vi "ImagerForFlowbit5_led.vi"() -> ()   [LabVIEW 2011]
uses:
  <vilib>/vision/Image Controls.llb/IMAQ Image.ctl
  <vilib>/Platform/TimedLoop/XDataNode/timing_clust.ctl
  <vilib>/Platform/TimedLoop/XDataNode/nitl_modes.ctl
  <vilib>/Platform/TimedLoop/XDataNode/wakeup.ctl
  <vilib>/Utility/config.llb/Read Key (I32).vi
  <vilib>/Analysis/1siggen.llb/Riffle Array (I32).vi
  <vilib>/Platform/TimedLoop/XDataNode/XDataNode.xnode
  <vilib>/Analysis/NI_AALBase.lvlib
  <vilib>/vision/NI_Vision_Development_Module.lvlib
  <vilib>/Platform/TimedLoop/XDataNode/XDNodeRunTimeDep.lvlib
  <vilib>/Utility/config.llb/NI_LVConfig.lvlib
panel:
  out "onLineMapOutput":T1[](array[typedef])
  out "Bounds.Right":i16
  out "停止循环":bool
  in  "Stimuli":i64=5
  in  "选项卡控件":enum32{"前面板", "参数设置", "OnLineMap"}(tab)
  out "log":string
  out "Stim_ID":i32(listbox)=1
  in  "开始/暂停":bool=TRUE
  in  "停止":bool
  out "重排的 Stim ID":i32[](array[numeric]) caption="重排的{X}"
  out "block":i32
  out "队列中元素数量":i32
  out "Image 2":T1(plugin-control)
  in  "热图":bool
  out "循环持续时间":i64
  out "Recording":bool
  out "grabLoop":i32
  out "writeing data":bool
  out "address":i16=888 caption="地址" format="%.0x"
  in  "SaveParameter":bool
  in  "Pra_binType":enum16{"Extract", "Resample"}(ring)
  in  "Pra_FramesPerStim":i64=16
  in  "Pra_Blk目录":path=path "D:/Expt/test"
  in  "Pra_文件名":string="G4_E02"
  in  "Pra_TimeForPrepare(ms)":u32=1000
  in  "Pra_stim ID":u8[](array[numeric])=[0, 2, 4, 6, 8]
  in  "Pra_blk总数":i32=500
  in  "Pra_stim protocol":T2(array[ring])=[enum."prep stim", enum."wait respirator", enum."show stim", enum."recording data", enum."Blank stim", enum."writing data", enum."ISI"]
  in  "Pra_blank stim":u8
  in  "Pra_wait（ms）":u32=10
  in  "Pra_ISI（ms）":u32=8000
  in  "Pra_FrameBin":i32=25
  in  "Pra_datatype":u16(ring)=13 items=["U8"=11, "I16"=12, "U32"=13, "SGL"=14]
  in  "FrameWidth":i64=704
  in  "FrameHeight":i64=576
  in  "LoadParameter":bool
  in  "Pra_bin":enum16{"1*1", "2*2"}(ring)
  in  "Pra_LED_Current(A)":dbl=0.5 min=0.0001 step=0.1
  in  "Pra_DR/R parameter":T3={"frame_zero_0"=0, "frame_zero_1"=1, "frame_0"=3, "frame_1"=15}
  in  "Pra_OnlineMap":cluster{"数组 1":i32[], "数组 2":i32[]}[](array[cluster])=[{"数组 1"=[2], "数组 2"=[6]}, {"数组 1"=[4], "数组 2"=[8]}, {"数组 1"=[2, 6], "数组 2"=[4, 8]}, {"数组 1"=[2, 4, 6, 8], "数组 2"=[0]}, {"数组 1"=[2, 4], "数组 2"=[6, 8]}]
  in  "Pra_clip ratio":dbl=2.0 min=0.0001 step=0.1
  in  "Pra_LED_COM":refnum<visa-resource-name>="COM3"
  in  "Pra_LED_Max_Voltage(V)":dbl=16.0
  # "-"
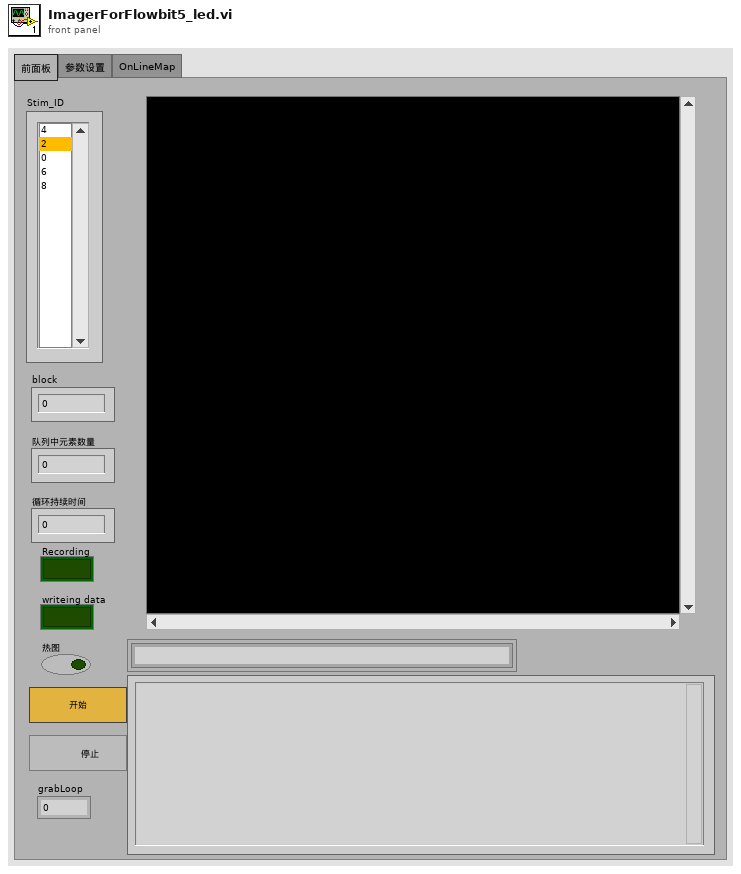
[diagram p1: front panel]
types:
  T1 = typedef "IMAQ Image.ctl" = refnum<image>
  T2 = enum16{"wait", "prep stim", "show stim", "wait respirator", "recording data", "Blank stim", "wait heart", "ISI", "DR/R", "wait calibrate", "openLightShutter", "closeLightShutter", "writing data", "LED on", "LED off"}[]
  T3 = cluster{"frame_zero_0":i32, "frame_zero_1":i32, "frame_0":i32, "frame_1":i32}
  T4 = typedef "Image Type" = u32
  T5 = enum16{"Disable External Trigger", "Enable External Trigger"}
  T6 = enum32{"Auto Detect", "RoadRunner", "Raven", "R64"}
  T7 = typedef "LVAllMonitorsDisplayTypeDef.ctl" = cluster{"Bounds":cluster{"Left":i16, "Top":i16, "Right":i16, "Bottom":i16}, "Depth":i16}[]
  T8 = cluster{"Bounds":cluster{"Left":i16, "Top":i16, "Right":i16, "Bottom":i16}, "Depth":i16}
  T9 = typedef "NI_LVConfig.lvlib/Config Data RefNum.ctl" = refnum<k1>
  T10 = enum16{"big-endian, network order", "native, host order", "little-endian"}
  T11 = enum8{"Enabled", "Disabled", "Disabled and Grayed Out"}
  T12 = enum16{"open", "replace", "create", "open or create", "replace or create", "replace or create with confirmation"}
  T13 = cluster{"Browser Size":cluster{"X":i32, "Y":i32}, "Images per Line":i32, "Background Color":u32, "Frame Size":i32, "Frame Style":enum16{"Raised", "Bevelled", "Outline", "Hidden", "Step", "Raised Outline"}}
  T14 = cluster{"Desired Font (Application)":enum16{"User-specified Font", "Application Font", "System Font", "Dialog Font"}, "[User-specified Font]":cluster{"Font Name":string, "Size":i16, "Strikeout?":bool, "Italic?":bool, "Underline?":bool, "Outline?":bool, "Shadow?":bool, "Bold?":bool, "Rotation Angle":dbl}, "Horizontal Alignment":i16, "Vertical Alignment":i16}
  T15 = typedef "XDNodeRunTimeDep.lvlib/timing_clust.ctl" = cluster{"Expected End [f-1]":u64, "Actual End [f-1]":u64, "Finished Late? [f-1]":bool, "Expected End [i-1]":u64, "Actual End [i-1]":u64, "Finished Late? [i-1]":bool, "Expected Start [i]":u64, "Actual Start [i]":u64, "Expected Start [f]":u64, "Actual Start [f]":u64, "Source Name":string, "Structure Name":string, "Period":i64, "Deadline":i64, "Offset":i64, "Start":i64, "Priority":i32, "Timeout":i32, "Mode":T16, "Wakeup Reason":T17, "Error":errorcluster, "Source Type":string, "Secondary Source Type":string, "Global End Time":u64, "Global Start Time":u64, "Frame Duration":u64, "Iteration Duration":u64, "Assigned CPU":i32, "I/O Scan Engine Mode":u32}
  T16 = typedef "XDNodeRunTimeDep.lvlib/nitl_modes.ctl" = enum32{"No Change", "Process missed periods, maintain original phase", "Discard missed periods, maintain original phase", "Process missed periods, ignore original phase", "Discard missed periods, ignore original phase"}
  T17 = typedef "XDNodeRunTimeDep.lvlib/wakeup.ctl" = enum32{"Normal", "Aborted", "Asynchronous wakeup", "Timing source error", "Timed loop error", "Timeout"}
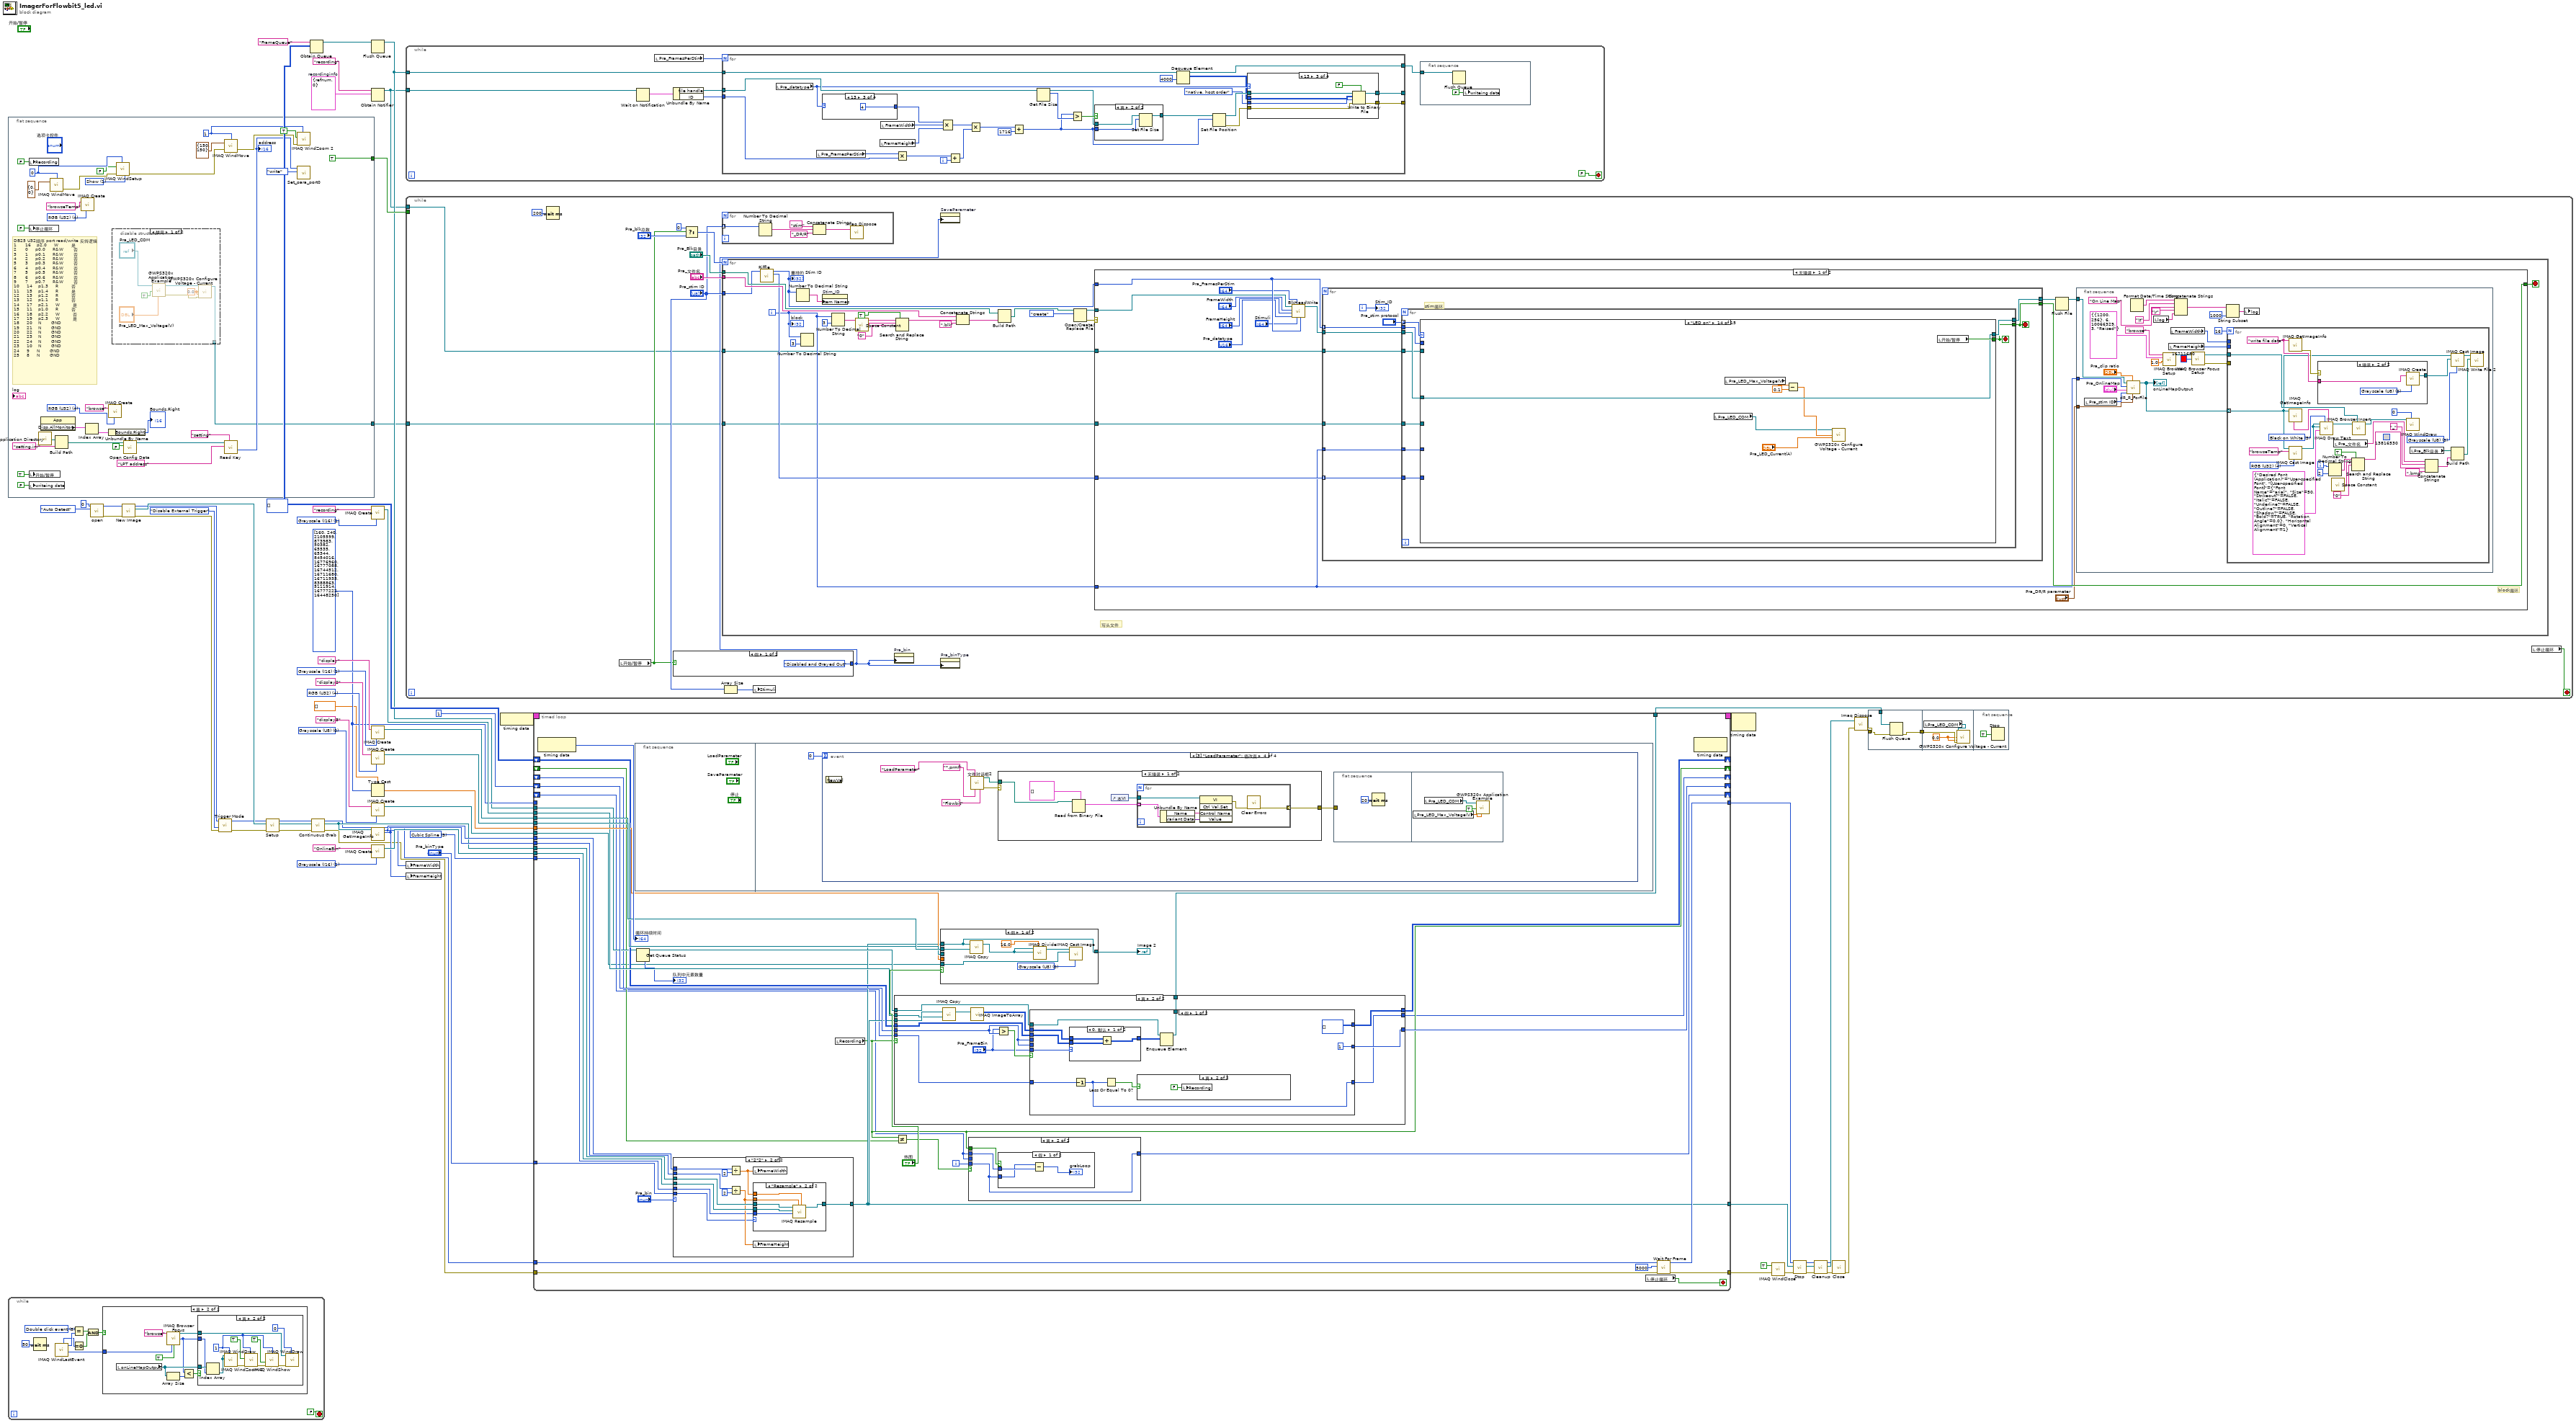
[diagram p0: block diagram]
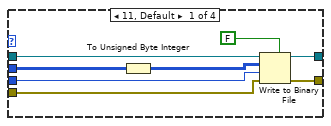
[diagram p4: hidden frame]
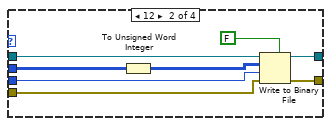
[diagram p5: hidden frame]
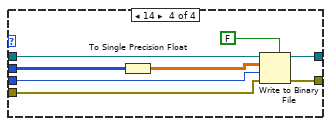
[diagram p6: hidden frame]
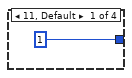
[diagram p8: hidden frame]
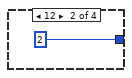
[diagram p9: hidden frame]
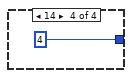
[diagram p10: hidden frame]
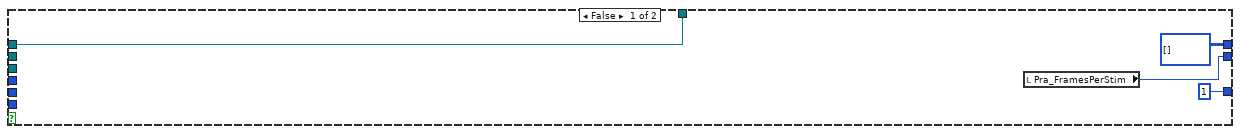
[diagram p11: hidden frame]
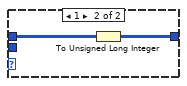
[diagram p13: hidden frame]
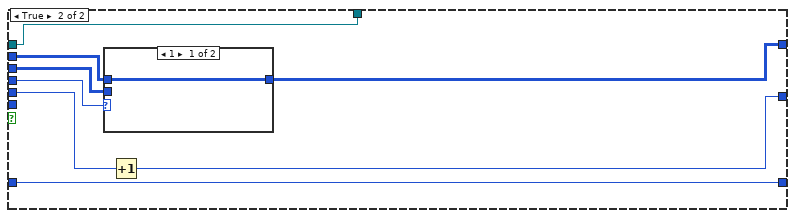
[diagram p14: hidden frame]
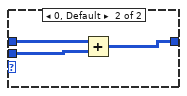
[diagram p15: hidden frame]
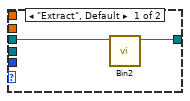
[diagram p19: hidden frame]
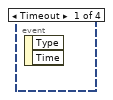
[diagram p20: hidden frame]
diagram:
  w11 = cluster{"file handle":refnum<file>, "ID":i32} {"file handle"=refnum, "ID"=0}  # recordinginfo
  w16 = T4 0 items=["Grayscale (U8)", "Grayscale (I16)", "Grayscale (SGL)", "Complex (CSG)", "RGB (U32)", "HSL (U32)", "RGB (U64)", "Grayscale (U16)"] ("Image Type")
  w21 = u32 3 items=["Zero Order", "Bi-Linear", "Quadratic", "Cubic Spline"] ("Interpolation Type")
  w23 = T4 1 items=["Grayscale (U8)", "Grayscale (I16)", "Grayscale (SGL)", "Complex (CSG)", "RGB (U32)", "HSL (U32)", "RGB (U64)", "Grayscale (U16)"] ("Image Type")
  w25 = u32[][] []
  w34 = T4 4 items=["Grayscale (U8)", "Grayscale (I16)", "Grayscale (SGL)", "Complex (CSG)", "RGB (U32)", "HSL (U32)", "RGB (U64)", "Grayscale (U16)"] ("Image Type")
  w32 = u32[] [160, 240, 2105599, 873983, 50382, 65535, 65344, 8454016, 16776960, 16777088, 16744512, 16711680, 16711935, 8388863, 5111914, 16777222, 16448250] ("数组")
  w38 = T4 1 items=["Grayscale (U8)", "Grayscale (I16)", "Grayscale (SGL)", "Complex (CSG)", "RGB (U32)", "HSL (U32)", "RGB (U64)", "Grayscale (U16)"] ("Image Type")
  w39 = T4 1 items=["Grayscale (U8)", "Grayscale (I16)", "Grayscale (SGL)", "Complex (CSG)", "RGB (U32)", "HSL (U32)", "RGB (U64)", "Grayscale (U16)"] ("Image Type")
  n1 = flat-sequence {
    tunnel: [TRUE ("Zoom to Fit Mode")] -> w27
    tunnel: [w66] -> w4
    frame #0 {
      w72 = 1 items=["Hide", "Show", "No change"] ("Scrollbars (No change)")
      w69 = 1 ("Window Number (0...15)")
      w73 = 0 ("Window Number (0...15)")
      w78 = T4 4 items=["Grayscale (U8)", "Grayscale (I16)", "Grayscale (SGL)", "Complex (CSG)", "RGB (U32)", "HSL (U32)", "RGB (U64)", "Grayscale (U16)"] ("Image Type")
      w79 = T4 4 items=["Grayscale (U8)", "Grayscale (I16)", "Grayscale (SGL)", "Complex (CSG)", "RGB (U32)", "HSL (U32)", "RGB (U64)", "Grayscale (U16)"] ("Image Type")
      # "DB25\tU32顺序\tport\tread/write\t反转逻辑\n1\t     16\t   p2.0    \tW\t        是\n2\t     0    \tp0.0\t   \tR&W\t      否\n3\t     1\t\t   p0.1\t   \tR&W      \t否\n4\t\t    2\t   \tp0.2   \t\tR&W      \t否\n5\t\t    3\t\t   p0.3   \t\tR&W\t      否\n6\t\t    4\t   \tp0.4   \t\tR&W      \t否\n7\t\t    5\t   \tp0.5   \t\tR&W      \t否\n8\t\t    6\t   \tp0.6\t   \tR&W      \t否\n9\t    \t7\t   \tp0.7\t   \tR&W\t      否\n10\t    14   \tp1.3   \t\tR        \t否\n11\t   \t15   \tp1.4   \t\tR        \t是\n12\t   \t13   \tp1.2\t   \tR        \t否\n13    \t12   \tp1.1\t   \tR        \t否\n14     17   \tp2.1\t   \tW        \t是\n15    \t11   \tp1.0   \t\tR\t        否\n16    \t18   \tp2.2   \t\tW        \t否\n17    \t19\t   p2.3   \t\tW\t        是\n18    \t20   \tN   \t  \tGND\t\n19    \t21   \tN   \t  \tGND\t\n20\t    22\t   N\t  \t  \tGND\t\n21\t    23\t   N  \t  \t\tGND\t\n22\t    24\t   N  \t  \t\tGND\t\n23    \t10   \tN  \t  \t\tGND\t\n24    \t9\t    N  \t  \t\tGND\t\n25\t    8    \tN  \t  \t\tGND"
      n2 = local write "Recording"(FALSE ("Recording")) -> ()
      n3 = local write "停止循环"(FALSE ("开始/暂停")) -> ()
      n4 = local write "开始/暂停"(TRUE ("开始/暂停")) -> ()
      n5 = local write "writeing data"(FALSE ("Recording")) -> ()
      n6 = call <vilib>:"Application Directory.vi"() -> ("Application Directory"=w91:path)
      n7 = property class="App"() -> ("Disp.AllMonitors"=w83:T7)  [unwired: 2 in, 2 out]
      n8 = call "IMAQ WindMove"("Window Number (0...15)"=w73, "Coordinates (screen)"=cluster{"X Position":i32, "Y Position":i32} {"X Position"=0, "Y Position"=0}) -> ("error out"=w74:errorcluster)  [unwired: 3 in, 1 out]
      n9 = Build Path(base path=w91, name or relative path="setting.ini" ("名称或相对路径")) -> (appended path=w89:path)
      n10 = call "IMAQ Create"("Image Name"="browseTemp", "Image Type"=w78) -> ()  [unwired: 3 in, 2 out]
      n11 = Index Array(array=w83) -> (element=w82:T8)  [unwired: 1 in]
      n12 = call "IMAQ Create"("Image Name"="browse", "Image Type"=w79) -> ()  [unwired: 3 in, 2 out]
      n13 = Unbundle By Name(w82) -> ("Bounds.Right"=→"Bounds.Right":i16)
      n14 = disable-structure shown="禁用" {
        disable-tunnel: [w100 _] -> w66
        frame Disabled {
          w101 = 0.0 ("Output Voltage (V) (0.0)")
          n15 = call <userlib>:"GWPS320x Application Example.vi"("OVP(V) (0.000)"="Pra_LED_Max_Voltage(V)", "Output State (F:Off)"=TRUE, "VISA session"="Pra_LED_COM") -> ("error out"=w99:errorcluster, "dup VISA session"=w102:refnum<visa-resource-name>)  [unwired: 5 in, 2 out]
          n16 = call <userlib>:"GWPS320x Configure Voltage - Current.vi"("VISA session"=w102, "Output Voltage (V) (0.0)"=w101, "Output Current (A) (0.0)"=w101, "error in (no error)"=w99) -> ("dup VISA session"=w100:refnum<visa-resource-name>)  [unwired: 10 in, 1 out]
        }
        frame Enabled {
        }
      }
      n17 = call "IMAQ WindSetup"("Scrollbars (No change)"=w72, "Window Number (0...15)"=w73, "error in (no error)"=w74, "Window can close? (Yes)"=FALSE) -> ("error out"=w71:errorcluster)  [unwired: 7 in]
      n18 = call <vilib>:"Open Config Data.vi"("create file if necessary (T)"=FALSE, "configuration file path"=w89) -> ("refnum"=w87:T9)  [unwired: 7 in, 2 out]
      n19 = call "IMAQ WindMove"("Window Number (0...15)"=w69, "Coordinates (screen)"=cluster{"X Position":i32, "Y Position":i32} {"X Position"=150, "Y Position"=150}, "error in (no error)"=w71) -> ("error out"=w70:errorcluster)  [unwired: 2 in, 1 out]
      n20 = call-poly <vilib>:"Read Key.vi"("section"="setting", "key"="LPT address", "refnum"=w87) -> ("value"=w84:i32)  [unwired: 5 in, 3 out]
      "address" <- w84
      n21 = call "IMAQ WindZoom 2"("Window Number (0...15)"=w69, "error in (no error)"=w70, "Zoom to Fit? (False)"=TRUE) -> ()  [unwired: 5 in, 4 out]
      n22 = call "Set_para_port0.vi"("R or W"=enum16{"read", "write"}."write", "address"=w84) -> ()  [unwired: 8 in, 2 out]
    }
  }
  n23 = while {
    stop <- FALSE stop-if-true
    w111 = 8 items=["No  event", "Click event", "Draw event", "Move event", "Size event", "Scroll event", "Activate event", "Close event", "Double click event"] ("Event")
    n24 = Wait (ms)(milliseconds to wait=u32 50 ("等待时间（毫秒）")) -> ()  [unwired: 1 out]
    n25 = call "IMAQ WindLastEvent"() -> ("Coordinates"=w105:i32[], "Event"=w110:i32, "Window Number (0...15)"=w109:i32)  [unwired: 6 in, 3 out]
    n26 = Equal?(x=w111, y=w110) -> (x = y?=w108:bool)
    n27 = Equal To 0?(x=w109) -> (x = 0?=w107:bool)
    n28 = And(x=w108, y=w107) -> (x .and. y?=w106:bool)
    n29 = case shown="真" w106 {
      tunnel: w105 -> [_ w121]
      frame False {
      }
      frame True {
        n30 = local read "onLineMapOutput"() -> (w117:T1[])
        n31 = call "IMAQ Browser Focus"("Image Browser In"="browse" ("Image Name"), "Pixel Position"=w121, "Get/Set (Set)"=TRUE) -> ("Image Browser Out"=w115:T1, "Index Out"=w116:i32)  [unwired: 5 in, 6 out]
        n32 = Array Size(array=w117) -> (size(s)=w119:i32)
        n33 = Less?(x=w116, y=w119) -> (x < y?=w118:bool)
        n34 = case shown="真" w118 {
          tunnel: w117 -> [_ w132]
          tunnel: w116 -> [_ w131]
          tunnel: w115 -> [_ w129]
          frame False {
          }
          frame True {
            w123 = 1 ("Window Number (0...15)")
            n35 = Index Array(array=w132, index=w131) -> (element=w130:T1)
            n36 = call "IMAQ WindDraw"("Window Number (0...15)"=w123, "Title"=w130, "Image"=w130) -> ("error out"=w126:errorcluster)  [unwired: 7 in, 1 out]
            n37 = call "IMAQ WindZoom 2"("Window Number (0...15)"=w123, "error in (no error)"=w126, "Zoom to Fit? (False)"=TRUE) -> ("error out"=w125:errorcluster)  [unwired: 5 in, 3 out]
            n38 = call "IMAQ WindShow"("error in (no error)"=w125, "Bring To Front? (N)"=TRUE, "Window Number (0...15)"=w123) -> ("error out"=w124:errorcluster)  [unwired: 3 in, 2 out]
            n39 = call "IMAQ WindDraw"("Window Number (0...15)"=0, "error in (no error)"=w124, "Image"=w129) -> ()  [unwired: 7 in, 2 out]
          }
        }
      }
    }
  }
  n40 = call <vilib>:"open.vi"("Board Type"=T6."Auto Detect", "Board Number"=u32 0) -> ("error out"=w53:errorcluster, "RefBrdOut"=w49:u32)  [unwired: 2 in, 5 out]
  n41 = call <vilib>:"New Image.vi"("RefBrdIn"=w49, "error in"=w53) -> ("RefBrdOut"=w48:u32, "Image"=w61:T1, "error out"=w54:errorcluster)  [unwired: 6 in]
  n42 = call <vilib>:"Trigger Mode.vi"("RefBrdIn"=w48, "Trigger Mode"=T5."Disable External Trigger", "error in (no error)"=w54) -> ("RefBrdOut"=w47:u32, "error out"=w55:errorcluster)  [unwired: 6 in]
  n43 = call <vilib>:"Setup.vi"("error in"=w55, "Image In"=w61, "RefBrdIn"=w47) -> ("error out"=w50:errorcluster, "Image"=w51:T1, "RefBrdOut"=w46:u32)  [unwired: 6 in]
  n44 = Obtain Queue(name (unnamed)="FrameQueue" ("名称（未命名）"), element data type=w25) -> (queue out=w28:refnum<queue>)  [unwired: 3 in, 2 out]
  n45 = call <vilib>:"Continuous Grab.vi"("error in (no error)"=w50, "Image In"=w51, "RefBrdIn"=w46) -> ("error out"=w5:errorcluster, "Image"=w17:T1, "RefBrdOut"=w6:u32)  [unwired: 6 in]
  n46 = Flush Queue(queue=w28) -> (queue out=w13:refnum<queue>)  [unwired: 1 in, 2 out]
  n47 = Obtain Notifier(name (unnamed)="recording" ("名称（未命名）"), notification data type=w11) -> (notifier out=w10:refnum<notifier>)  [unwired: 2 in, 2 out]
  n48 = call "IMAQ Create"("Image Name"="recording", "Image Type"=w39) -> ("New Image"=w41:T1)  [unwired: 3 in, 1 out]
  n49 = call "IMAQ Create"("Image Name"="display", "Image Type"=w38) -> ("New Image"=w36:T1)  [unwired: 3 in, 1 out]
  n50 = call "IMAQ Create"("Image Name"="display2", "Image Type"=w34) -> ("New Image"=w33:T1)  [unwired: 3 in, 1 out]
  n51 = Type Cast(type=sgl[] [] ("单精度浮点"), x=w32) -> (*(type *) &x=w30:sgl[])
  n52 = call "IMAQ Create"("Image Name"="display3", "Image Type"=w16) -> ("New Image"=w14:T1)  [unwired: 3 in, 1 out]
  n53 = call "IMAQ GetImageInfo"("Image"=w17) -> ("Y Resolution"=w19:i32, "X Resolution"=w20:i32)  [unwired: 3 in, 6 out]
  n54 = call "IMAQ Create"("Image Name"="OnlineBin", "Image Type"=w23) -> ("New Image"=w22:T1)  [unwired: 3 in, 1 out]
  n55 = while {
    tunnel: w13 -> [w139]
    tunnel: w10 -> [w137]
    stop <- FALSE stop-if-true
    n56 = Wait on Notification(notifier=w137) -> (notification=w136:cluster{"file handle":refnum<file>, "ID":i32})  [unwired: 3 in, 3 out]
    n57 = local read "Pra_FramesPerStim"() -> (w138:i64)
    n58 = Unbundle By Name(w136) -> ("file handle"=w135:refnum<file>, "ID"=w134:i32)
    n59 = for {
      N: w138 -> [_]
      tunnel: w135 -> [w169]
      tunnel: w134 -> [w153]
      tunnel: [w161] -> _
      tunnel: [w160] -> w133
      tunnel: w139 -> [w145]
      tunnel: [w143] -> _
      i -> [w151]
      n60 = local read "Pra_datatype"() -> (w165:u16)
      n61 = local read "Pra_FramesPerStim"() -> (w154:i64)
      n62 = case shown="13" w165 {
        tunnel: [i64 1 i64 2 i64 4 i64 4] -> w157
        frame 11, Default {
        }
        frame 12 {
        }
        frame 13 {
        }
        frame 14 {
        }
      }
      n63 = local read "FrameHeight"() -> (w155:i64)
      n64 = local read "FrameWidth"() -> (w156:i64)
      n65 = Multiply(x=w154, y=w153) -> (x*y=w152:i64)
      n66 = Compound Arithmetic op=MULTIPLY(w157, w156, w155) -> (w149:i64)
      n67 = Add(x=w152, y=w151) -> (x+y=w150:i64)
      n68 = Multiply(x=w149, y=w150) -> (x*y=w148:i64)
      n69 = Add(x=w148, y=i64 1716 ("x")) -> (x+y=w146:i64)
      n70 = Get File Size(file=w169) -> (refnum out=w162:refnum<file>, size (in bytes)=w158:i64)  [unwired: 1 in, 1 out]
      n71 = Greater?(x=w146, y=w158) -> (0:w163:bool)
      n72 = case shown="真" w163 {
        tunnel: w146 -> [_ w204]
        tunnel: w162 -> [w201 w203]
        tunnel: [w201 w202] -> w164
        frame False {
        }
        frame True {
          n73 = Set File Size(6:w204, 7:w203) -> (3:w202:refnum<file>)  [unwired: 1 in, 1 out]
        }
      }
      n74 = Dequeue Element(queue=w145, timeout in ms (-1)=4000 ("超时毫秒(-1)")) -> (queue out=w160:refnum<queue>, element=w144:u32[][])  [unwired: 1 in, 2 out]
      n75 = Set File Position(offset (in bytes) (0)=w146, refnum=w164) -> (refnum out=w168:refnum<file>, error out=w166:errorcluster)  [unwired: 2 in]
      n76 = case shown="13" w165 {
        tunnel: w144 -> [w172 w181 w187 w194]
        tunnel: w168 -> [w176 w182 w190 w196]
        tunnel: T10."native, host order" ("字节顺序(0:big-endian, network order)") -> [w175 w183 w188 w197]
        tunnel: w166 -> [w174 w178 w189 w198]
        tunnel: [w173 w184 w191 w199] -> w161
        tunnel: [w170 w179 w186 w193] -> w143
        frame 11, Default {
          n77 = To Unsigned Byte Integer(number=w172) -> (unsigned 8bit integer=w171:u8[][])
          n78 = Write to Binary File(file (use dialog)=w176, data=w171, error in=w174, 5:FALSE ("预置数组或字符串大小？(T)"), 9:w175) -> (refnum out=w173:refnum<file>, error out=w170:errorcluster)  [unwired: 1 in, 1 out]
        }
        frame 12 {
          n79 = To Unsigned Word Integer(number=w181) -> (unsigned 16bit integer=w180:u16[][])
          n80 = Write to Binary File(file (use dialog)=w182, data=w180, error in=w178, 5:FALSE ("预置数组或字符串大小？(T)"), 9:w183) -> (refnum out=w184:refnum<file>, error out=w179:errorcluster)  [unwired: 1 in, 1 out]
        }
        frame 13 {
          n81 = Write to Binary File(file (use dialog)=w190, data=w187, error in=w189, 5:FALSE ("预置数组或字符串大小？(T)"), 9:w188) -> (refnum out=w191:refnum<file>, error out=w186:errorcluster)  [unwired: 1 in, 1 out]
        }
        frame 14 {
          n82 = To Single Precision Float(number=w194) -> (single precision float=w195:sgl[][])
          n83 = Write to Binary File(file (use dialog)=w196, data=w195, error in=w198, 5:FALSE ("预置数组或字符串大小？(T)"), 9:w197) -> (refnum out=w199:refnum<file>, error out=w193:errorcluster)  [unwired: 1 in, 1 out]
        }
      }
    }
    n84 = flat-sequence {
      tunnel: w133 -> [w142]
      frame #0 {
        n85 = Flush Queue(queue=w142) -> ()  [unwired: 1 in, 3 out]
        n86 = local write "writeing data"(FALSE ("writeing data")) -> ()
      }
    }
  }
  n87 = while {
    tunnel: w27 -> [_]
    tunnel: w10 -> [w210]
    tunnel: w4 -> [w209]
    stop <- w220 stop-if-true
    n88 = Wait (ms)(milliseconds to wait=u32 200 ("等待时间（毫秒）")) -> ()  [unwired: 1 out]
    n89 = local read "开始/暂停"() -> (w212:bool)
    n90 = case shown="假" w212 {
      tunnel: [T11."Disabled and Grayed Out" ("禁用") T11."Enabled" ("禁用")] -> w211
      frame False {
      }
      frame True {
      }
    }
    n91 = Select(t=0, s=w212, f="Pra_blk总数") -> (s? t:f=w217:i32)
    n92 = for {
      tunnel: "Pra_stim ID" -> [w225] mode=indexing
      n93 = Number To Decimal String(number=w225) -> (decimal integer string=w226:string)  [unwired: 1 in]
      n94 = Concatenate Strings("stim" ("字符串"), w226, "_DR/R" ("字符串")) -> (w224:string)
      n95 = call "Imaq Dispose"("Image"=w224) -> ()  [unwired: 5 in, 1 out]
    }
    n96 = for {
      N: w217 -> [_]
      tunnel: "Pra_stim ID" -> [w247]
      tunnel: "Pra_文件名" -> [w251]
      tunnel: "Pra_Blk目录" -> [w250]
      tunnel: w210 -> [w243]
      tunnel: w209 -> [w229]
      i -> [w245]
      stop <- w248 stop-if-true
      # "写头文件"
      n97 = call-poly <vilib>:"Riffle.vi"("X"=w247) -> ("Riffled Index"=w246:i32[], "Riffled {X}"=w249:i32[])  [unwired: 8 in, 1 out]
      "重排的 Stim ID" <- w249
      n98 = Number To Decimal String(number=w249) -> (decimal integer string=w233:string[])  [unwired: 1 in]
      n99 = Number To Decimal String(number=w245, width (-)=i16 3 ("宽度(-)")) -> ()  [unwired: 1 out]
      n100 = property on="Stim_ID" class="LstBox (严格)"("Item Names"=w233) -> ()  [unwired: 2 in, 2 out]
      n101 = Number To Decimal String(number=w245, width (-)=i16 3 ("宽度(-)")) -> (decimal integer string=w238:string)
      n102 = call <vilib>:"Space Constant.vi"() -> ("String"=w239:string)
      n103 = Search and Replace String(replace all?=TRUE ("替换全部？(F)"), input string=w238, search string=w239, replace string="0" ("替换字符串(\"\")")) -> (result string=w236:string)  [unwired: 4 in, 3 out]
      n104 = Concatenate Strings(w251, w236, ".blk" ("字符串")) -> (w234:string)
      n105 = Build Path(base path=w250, name or relative path=w234) -> (appended path=w244:path)
      n106 = Open/Create/Replace File(file path (use dialog)=w244, operation (0:open)=T12."create" ("操作(0:open)")) -> (refnum out=w231:refnum<file>, error out=w230:errorcluster)  [unwired: 4 in, 1 out]
      n107 = case shown="无错误" w230 {
        tunnel: w249 -> [w266 _]
        tunnel: [w265 TRUE ("开始/暂停")] -> w248
        tunnel: w246 -> [w264 _]
        tunnel: w245 -> [w262 _]
        tunnel: w243 -> [w259 _]
        tunnel: w231 -> [w254 _]
        tunnel: w229 -> [w252 _]
        frame No Error {
          # "block循环"
          n108 = call "BlkHeadWrite.vi"("SequenceOfID"=w266, "Stimuli"="Stimuli", "FramesPerStim"="Pra_FramesPerStim", "datatype"="Pra_datatype", "FrameHeight"="FrameHeight", "FrameWidth"="FrameWidth", "引用句柄输入"=w254) -> ("引用句柄输出"=w267:refnum<file>)  [unwired: 4 in]
          n109 = for {
            tunnel: w267 -> [w335]
            tunnel: [w333] -> w261
            tunnel: w264 -> [w334] mode=indexing
            tunnel: w266 -> [w332] mode=indexing
            tunnel: [w331] -> w265
            tunnel: w262 -> [w328]
            tunnel: w259 -> [w327]
            tunnel: w252 -> [w326]
            i -> [w330]
            stop <- w331 stop-if-true
            # "stim循环"
            n110 = for {
              tunnel: w334 -> [w343]
              tunnel: w332 -> [w341]
              tunnel: [w339] -> w331
              tunnel: "Pra_stim protocol" -> [w340] mode=indexing
              tunnel: w335 -> [w344]
              tunnel: [w342] -> w333
              tunnel: w328 -> [w338]
              tunnel: w327 -> [w337]
              tunnel: w326 -> [w336]
              stop <- w339 stop-if-true
              n111 = case shown="\"LED on\"" w340 {
                tunnel: w344 -> [w347 w367 w382 w396 w413 w426 w440 w455 w477 w487 w489 w502 w515 w531 w539]
                tunnel: w343 -> [_ _ _ w398 _ _ _ w453 _ _ _ _ _ _ _]
                tunnel: [w347 w367 w382 w396 w413 w426 w440 w455 w477 w487 w489 w502 w515 w531 w539] -> w342
                tunnel: w341 -> [w345 _ _ _ _ _ _ _ _ _ _ _ _ _ _]
                tunnel: [w348 w368 w383 w395 w414 w427 w441 w454 w478 w488 w490 w503 w516 w532 w540] -> w339
                tunnel: w338 -> [_ _ _ _ _ _ _ w452 _ _ _ _ _ _ _]
                tunnel: w337 -> [_ _ _ w399 _ _ _ _ _ _ _ _ _ _ _]
                tunnel: w336 -> [_ _ _ _ _ _ _ _ _ _ _ _ _ _ w534]
                frame "prep stim" {
                  n112 = Number To Boolean Array(number=w345) -> (Boolean array=w349:bool[])
                  n113 = flat-sequence {
                    tunnel: w349 -> [w360]
                    tunnel: [w360] -> w346
                    tunnel: w345 -> [w359]
                    tunnel: w346 -> [w365]
                    frame #0 {
                      n114 = Number To Decimal String(number=w359) -> (decimal integer string=w356:string)  [unwired: 1 in]
                      n115 = Format Date/Time String() -> (date/time string=w358:string)  [unwired: 3 in]
                      n116 = local read "log"() -> (w352:string)
                      n117 = Concatenate Strings(w358, "\t", "prep stim ID=" ("字符串"), w356, "\r", w352) -> (w354:string)
                      n118 = String Subset(string=w354, length (rest)=1000 ("y")) -> (substring=w353:string)  [unwired: 1 in]
                      n119 = local write "log"(w353) -> ()
                    }
                    frame #1 {
                      n120 = local read "address"() -> (w362:i16)
                      n121 = local read "address"() -> (w361:i16)
                      n122 = call "Write_para_port0.vi"("port0（8元素）"=w365, "address"=w361) -> ()  [unwired: 9 in, 1 out]
                      n123 = call "Write_para_port2_singalChange.vi"("索引"=0, "布尔"=TRUE, "address"=w362) -> ()  [unwired: 8 in, 1 out]
                    }
                    frame #2 {
                      n124 = Wait (ms)(milliseconds to wait="Pra_TimeForPrepare(ms)") -> ()  [unwired: 1 out]
                    }
                  }
                  n125 = local read "开始/暂停"() -> (w348:bool)
                }
                frame "wait respirator" {
                  n126 = while {
                    stop <- w379 stop-if-true
                    # "this step will return true if pallel port doesn't connect any signal.That means this loop only run once."
                    n127 = Wait (ms)(milliseconds to wait=u32 5 ("等待时间（毫秒）")) -> ()  [unwired: 1 out]
                    n128 = local read "address"() -> (w377:i16)
                    n129 = call "read_para_port1.vi"("address"=w377) -> ("port1（5元素）"=w381:bool[])  [unwired: 9 in, 1 out]
                    n130 = Index Array(array=w381, index=3 ("索引")) -> (element=w379:bool)
                  }
                  n131 = flat-sequence {
                    frame #0 {
                      n132 = Format Date/Time String() -> (date/time string=w376:string)  [unwired: 3 in]
                      n133 = local read "log"() -> (w371:string)
                      n134 = Concatenate Strings(w376, "\t", "wait respiratory" ("字符串"), "\r", w371) -> (w373:string)
                      n135 = String Subset(string=w373, length (rest)=1000 ("y")) -> (substring=w372:string)  [unwired: 1 in]
                      n136 = local write "log"(w372) -> ()
                    }
                  }
                  n137 = local read "开始/暂停"() -> (w368:bool)
                }
                frame "show stim" {
                  n138 = flat-sequence {
                    frame #0 {
                      n139 = local read "address"() -> (w392:i16)
                      n140 = call "Write_para_port2_singalChange.vi"("索引"=0, "布尔"=FALSE, "address"=w392) -> ()  [unwired: 8 in, 1 out]
                    }
                  }
                  n141 = flat-sequence {
                    frame #0 {
                      n142 = Format Date/Time String() -> (date/time string=w391:string)  [unwired: 3 in]
                      n143 = local read "log"() -> (w386:string)
                      n144 = Concatenate Strings(w391, "\t", "show stim" ("字符串"), "\r", w386) -> (w388:string)
                      n145 = String Subset(string=w388, length (rest)=1000 ("y")) -> (substring=w387:string)  [unwired: 1 in]
                      n146 = local write "log"(w387) -> ()
                    }
                  }
                  n147 = local read "开始/暂停"() -> (w383:bool)
                }
                frame "recording data" {
                  n148 = flat-sequence {
                    frame #0 {
                      n149 = Format Date/Time String() -> (date/time string=w411:string)  [unwired: 3 in]
                      n150 = local read "log"() -> (w406:string)
                      n151 = Concatenate Strings(w411, "\t", "recording data" ("字符串"), "\r", w406) -> (w408:string)
                      n152 = String Subset(string=w408, length (rest)=1000 ("y")) -> (substring=w407:string)  [unwired: 1 in]
                      n153 = local write "log"(w407) -> ()
                    }
                  }
                  n154 = flat-sequence {
                    frame #0 {
                      "Recording" <- TRUE ("Recording")
                      "writeing data" <- TRUE ("Recording")
                    }
                    frame #1 {
                      n155 = while {
                        stop <- w403 continue-if-true
                        n156 = local read "Recording"() -> (w403:bool)
                        n157 = Wait (ms)(milliseconds to wait=u32 1 ("等待时间（毫秒）")) -> ()  [unwired: 1 out]
                      }
                    }
                  }
                  n158 = Bundle("引用句柄输出"=w396, w398) -> (w397:cluster{"引用句柄输出":refnum<file>, i32})  [unwired: 1 in]
                  n159 = Send Notification(notification=w397, notifier=w399) -> ()  [unwired: 1 in, 2 out]
                  n160 = local read "开始/暂停"() -> (w395:bool)
                }
                frame "Blank stim" {
                  n161 = flat-sequence {
                    frame #0 {
                      n162 = Format Date/Time String() -> (date/time string=w424:string)  [unwired: 3 in]
                      n163 = local read "log"() -> (w419:string)
                      n164 = Concatenate Strings(w424, "\t", "show blank stim" ("字符串"), "\r", w419) -> (w421:string)
                      n165 = String Subset(string=w421, length (rest)=1000 ("y")) -> (substring=w420:string)  [unwired: 1 in]
                      n166 = local write "log"(w420) -> ()
                    }
                  }
                  n167 = local read "address"() -> (w412:i16)
                  n168 = Number To Boolean Array(number="Pra_blank stim") -> (Boolean array=w415:bool[])
                  n169 = call "Write_para_port0.vi"("port0（8元素）"=w415, "address"=w412) -> ()  [unwired: 9 in, 1 out]
                  n170 = local read "开始/暂停"() -> (w414:bool)
                }
                frame "ISI" {
                  n171 = flat-sequence {
                    tunnel: "Pra_ISI（ms）" -> [w431]
                    tunnel: "Pra_ISI（ms）" -> [w438]
                    frame #0 {
                      n172 = Number To Decimal String(number=w431) -> (decimal integer string=w435:string)  [unwired: 1 in]
                      n173 = Format Date/Time String() -> (date/time string=w437:string)  [unwired: 3 in]
                      n174 = local read "log"() -> (w430:string)
                      n175 = Concatenate Strings(w437, "\t", "ISI(ms)=" ("字符串"), w435, "\r", w430) -> (w433:string)
                      n176 = String Subset(string=w433, length (rest)=1000 ("y")) -> (substring=w432:string)  [unwired: 1 in]
                      n177 = local write "log"(w432) -> ()
                    }
                    frame #1 {
                      n178 = Wait (ms)(milliseconds to wait=w438) -> ()  [unwired: 1 out]
                    }
                  }
                  n179 = local read "开始/暂停"() -> (w427:bool)
                }
                frame "wait", Default {
                  n180 = Wait (ms)(milliseconds to wait="Pra_wait（ms）") -> ()  [unwired: 1 out]
                  n181 = flat-sequence {
                    tunnel: "Pra_wait（ms）" -> [w445]
                    frame #0 {
                      n182 = Number To Decimal String(number=w445) -> (decimal integer string=w449:string)  [unwired: 1 in]
                      n183 = Format Date/Time String() -> (date/time string=w451:string)  [unwired: 3 in]
                      n184 = local read "log"() -> (w444:string)
                      n185 = Concatenate Strings(w451, "\t", "wait(ms)=" ("字符串"), w449, "\r", w444) -> (w447:string)
                      n186 = String Subset(string=w447, length (rest)=1000 ("y")) -> (substring=w446:string)  [unwired: 1 in]
                      n187 = local write "log"(w446) -> ()
                    }
                  }
                  n188 = local read "开始/暂停"() -> (w441:bool)
                }
                frame "DR/R" {
                  n189 = disable-structure shown="禁用" {
                    frame Disabled {
                      n190 = flat-sequence {
                        frame #0 {
                          n191 = Format Date/Time String() -> (date/time string=w463:string)  [unwired: 3 in]
                          n192 = local read "log"() -> (w458:string)
                          n193 = Concatenate Strings(w463, "\t", "DR/R" ("字符串"), "\r", w458) -> (w460:string)
                          n194 = String Subset(string=w460, length (rest)=1000 ("y")) -> (substring=w459:string)  [unwired: 1 in]
                          n195 = local write "log"(w459) -> ()
                        }
                      }
                    }
                    frame Enabled {
                    }
                  }
                  n196 = disable-structure shown="禁用" {
                    disable-tunnel: w453 -> [w468 _]
                    disable-tunnel: w452 -> [w467 _]
                    frame Disabled {
                      n197 = local read item#-1() -> (w464)
                      n198 = Index Array(array=w464, index=w468) -> (element=w465)
                      n199 = call "dR.vi"() -> ("Image Dst Out"=w466:T1)  [unwired: 11 in]
                      n200 = case shown="0" w467 {
                        selector: w467 -> [_ w473]
                        tunnel: w466 -> [w470 w474]
                        tunnel: w465 -> [w469 w476]
                        frame 0 {
                          n201 = call "IMAQ Copy"("Image Dst"=w469, "Image Src"=w470) -> ()  [unwired: 4 in, 2 out]
                        }
                        frame 1, Default {
                          n202 = Increment(x=w473) -> (x+1=w472:i32)
                          n203 = call "IMAQ Multiply"("Image Src A"=w476, "Constant"=w473, "Image Dst"=w476) -> ("Image Dst Out"=w475:T1)  [unwired: 4 in, 1 out]
                          n204 = call "IMAQ Add"("Image Src A"=w475, "Image Dst"=w475, "Image Src B"=w474) -> ("Image Dst Out"=w471:T1)  [unwired: 4 in, 1 out]
                          n205 = call "IMAQ Divide"("Image Src A"=w471, "Constant"=w472, "Image Dst"=w471) -> ()  [unwired: 4 in, 2 out]
                        }
                      }
                    }
                    frame Enabled {
                    }
                  }
                  n206 = local read "开始/暂停"() -> (w454:bool)
                }
                frame "wait heart" {
                  n207 = flat-sequence {
                    frame #0 {
                      n208 = Format Date/Time String() -> (date/time string=w486:string)  [unwired: 3 in]
                      n209 = local read "log"() -> (w481:string)
                      n210 = Concatenate Strings(w486, "\t", "wait heart" ("字符串"), "\r", w481) -> (w483:string)
                      n211 = String Subset(string=w483, length (rest)=1000 ("y")) -> (substring=w482:string)  [unwired: 1 in]
                      n212 = local write "log"(w482) -> ()
                    }
                  }
                  n213 = local read "开始/暂停"() -> (w478:bool)
                }
                frame "wait calibrate" {
                  n214 = local read "开始/暂停"() -> (w488:bool)
                }
                frame "openLightShutter" {
                  n215 = flat-sequence {
                    frame #0 {
                      n216 = local read "address"() -> (w499:i16)
                      n217 = call "Write_para_port2_singalChange.vi"("索引"=1, "布尔"=TRUE, "address"=w499) -> ()  [unwired: 8 in, 1 out]
                    }
                  }
                  n218 = flat-sequence {
                    frame #0 {
                      n219 = Format Date/Time String() -> (date/time string=w498:string)  [unwired: 3 in]
                      n220 = local read "log"() -> (w493:string)
                      n221 = Concatenate Strings(w498, "\t", "open light shutter" ("字符串"), "\r", w493) -> (w495:string)
                      n222 = String Subset(string=w495, length (rest)=1000 ("y")) -> (substring=w494:string)  [unwired: 1 in]
                      n223 = local write "log"(w494) -> ()
                    }
                  }
                  n224 = local read "开始/暂停"() -> (w490:bool)
                }
                frame "closeLightShutter" {
                  n225 = flat-sequence {
                    frame #0 {
                      n226 = local read "address"() -> (w512:i16)
                      n227 = call "Write_para_port2_singalChange.vi"("索引"=1, "布尔"=FALSE, "address"=w512) -> ()  [unwired: 8 in, 1 out]
                    }
                  }
                  n228 = flat-sequence {
                    frame #0 {
                      n229 = Format Date/Time String() -> (date/time string=w511:string)  [unwired: 3 in]
                      n230 = local read "log"() -> (w506:string)
                      n231 = Concatenate Strings(w511, "\t", "close light shutter" ("字符串"), "\r", w506) -> (w508:string)
                      n232 = String Subset(string=w508, length (rest)=1000 ("y")) -> (substring=w507:string)  [unwired: 1 in]
                      n233 = local write "log"(w507) -> ()
                    }
                  }
                  n234 = local read "开始/暂停"() -> (w503:bool)
                }
                frame "writing data" {
                  n235 = while {
                    stop <- w525 continue-if-true
                    n236 = local read "writeing data"() -> (w525:bool)
                    n237 = Wait (ms)(milliseconds to wait=u32 1 ("等待时间（毫秒）")) -> ()  [unwired: 1 out]
                  }
                  n238 = flat-sequence {
                    frame #0 {
                      n239 = Format Date/Time String() -> (date/time string=w524:string)  [unwired: 3 in]
                      n240 = local read "log"() -> (w519:string)
                      n241 = Concatenate Strings(w524, "\t", "writing data" ("字符串"), "\r", w519) -> (w521:string)
                      n242 = String Subset(string=w521, length (rest)=1000 ("y")) -> (substring=w520:string)  [unwired: 1 in]
                      n243 = local write "log"(w520) -> ()
                    }
                  }
                  n244 = local read "开始/暂停"() -> (w516:bool)
                }
                frame "LED on" {
                  n245 = local read "Pra_LED_COM"() -> (w527:refnum<visa-resource-name>)
                  n246 = local read "Pra_LED_Max_Voltage(V)"() -> (w530:dbl)
                  n247 = Subtract(x=w530, y=0.1) -> (x-y=w528:dbl)
                  n248 = call <userlib>:"GWPS320x Configure Voltage - Current.vi"("VISA session"=w527, "Output Voltage (V) (0.0)"=w528, "Output Current (A) (0.0)"="Pra_LED_Current(A)") -> ()  [unwired: 11 in, 2 out]
                  n249 = local read "开始/暂停"() -> (w532:bool)
                }
                frame "LED off" {
                  n250 = local read "Pra_LED_Max_Voltage(V)"() -> (w537:dbl)
                  n251 = Subtract(x=w537, y=0.1) -> (x-y=w535:dbl)
                  n252 = call <userlib>:"GWPS320x Configure Voltage - Current.vi"("VISA session"=w534, "Output Voltage (V) (0.0)"=w535, "Output Current (A) (0.0)"=0.0 ("Pra_LED_Current(A) 2")) -> ()  [unwired: 11 in, 2 out]
                  n253 = local read "开始/暂停"() -> (w540:bool)
                }
              }
            }
            "Stim_ID" <- w330
          }
          n254 = Flush File(refnum=w261) -> (refnum out=w260:refnum<file>)  [unwired: 1 in, 1 out]
          n255 = flat-sequence {
            tunnel: "Pra_DR/R parameter" -> [w292]
            tunnel: w260 -> [w291]
            tunnel: w262 -> [w290]
            frame #0 {
              n256 = local read "Pra_stim ID"() -> (w289:u8[])
              n257 = call "dR_R_ForFile.vi"("DR/R parameter"=w292, "clip ratio"="Pra_clip ratio", "stim ID"=w289, "OnlineMap"="Pra_OnlineMap", "blkIndex"=w290, "BlkFile"=w291) -> ("onLineMapOutput"=w287:T1[])  [unwired: 5 in]
              "onLineMapOutput" <- w287
              n258 = Format Date/Time String() -> (date/time string=w286:string)  [unwired: 3 in]
              n259 = local read "log"() -> (w281:string)
              n260 = call "IMAQ Browser Setup"("Image Ratio"=sgl 1.0, "Browser Info"=T13 {"Browser Size"={"X"=1200, "Y"=256}, "Images per Line"=6, "Background Color"=10066329, "Frame Size"=3, "Frame Style"=enum."Raised"}, "Image In"="browse" ("Image Name")) -> ("Image Browser Out"=w272:T1)  [unwired: 1 in, 3 out]
              n261 = local read "FrameHeight"() -> (w277:i64)
              n262 = local read "FrameWidth"() -> (w278:i64)
              n263 = Concatenate Strings(w286, "\t", "On Line Map" ("字符串"), "\r", w281) -> (w283:string)
              n264 = call "IMAQ Browser Focus Setup"("Focus Color"=u32 16711680, "Image Browser In"=w272) -> ("error out"=w268:errorcluster, "Image Browser Out"=w271:T1)  [unwired: 2 in]
              n265 = String Subset(string=w283, length (rest)=1000 ("y")) -> (substring=w282:string)  [unwired: 1 in]
              n266 = for {
                N: 16 -> [_]
                tunnel: w287 -> [w299] mode=indexing
                tunnel: w278 -> [_]
                tunnel: w277 -> [_]
                tunnel: w271 -> [w304]
                tunnel: w268 -> [_]
                i -> [w305]
                w296 = 3 items=["White", "Black", "Inverted", "Black on White", "White on Black"] ("Color")
                (unwired) u32 13816530 ("BG Color (Transparent)")
                w301 = T4 4 items=["Grayscale (U8)", "Grayscale (I16)", "Grayscale (SGL)", "Complex (CSG)", "RGB (U32)", "HSL (U32)", "RGB (U64)", "Grayscale (U16)"] ("Image Type")
                w307 = "write file data" ("替换字符串(\"\")")
                w310 = T4 0 items=["Grayscale (U8)", "Grayscale (I16)", "Grayscale (SGL)", "Complex (CSG)", "RGB (U32)", "HSL (U32)", "RGB (U64)", "Grayscale (U16)"] ("Image Type")
                n267 = call "IMAQ GetImageInfo"("Image"=w299) -> ("Image Name"=w295:string)  [unwired: 3 in, 7 out]
                n268 = call "IMAQ Cast Image"("Image Type"=w301, "Image Dst"="browseTemp" ("Image Name"), "Image Src"=w299) -> ("Image Dst Out"=w298:T1)  [unwired: 7 in, 1 out]
                n269 = call "IMAQ GetImageInfo"("Image"=w307) -> ("error out"=w308:errorcluster)  [unwired: 3 in, 7 out]
                n270 = case shown="错误" w308 {
                  tunnel: w307 -> [w322 w324]
                  tunnel: [w322 w323] -> w306
                  frame No Error {
                  }
                  frame Error {
                    w325 = T4 0 items=["Grayscale (U8)", "Grayscale (I16)", "Grayscale (SGL)", "Complex (CSG)", "RGB (U32)", "HSL (U32)", "RGB (U64)", "Grayscale (U16)"] ("Image Type")
                    n271 = call "IMAQ Create"("Image Name"=w324, "Image Type"=w325) -> ("New Image"=w323:T1)  [unwired: 3 in, 1 out]
                  }
                }
                n272 = call "IMAQ Draw Text"("String"=w295, "Color"=w296, "Font, Size & Style"=T14 {"Desired Font (Application)"=enum."User-specified Font", "[User-specified Font]"={"Font Name"="arial", "Size"=50, "Strikeout?"=FALSE, "Italic?"=FALSE, "Underline?"=FALSE, "Outline?"=FALSE, "Shadow?"=FALSE, "Bold?"=TRUE, "Rotation Angle"=0.0}, "Horizontal Alignment"=0, "Vertical Alignment"=1}, "Image Dst"=w298, "Image Src"=w298) -> ("Image Dst Out"=w294:T1)  [unwired: 3 in, 3 out]
                n273 = Number To Decimal String(number=w305, width (-)=i16 2 ("宽度(-)")) -> (decimal integer string=w319:string)
                n274 = call <vilib>:"Space Constant.vi"() -> ("String"=w318:string)
                n275 = local read "Pra_文件名"() -> (w321:string)
                n276 = Search and Replace String(replace all?=TRUE ("替换全部？(F)"), input string=w319, search string=w318, replace string="0" ("替换字符串(\"\")")) -> (result string=w314:string)  [unwired: 4 in, 3 out]
                n277 = call "IMAQ Browser Insert"("Image Browser In"=w304, "Image to Add"=w294) -> ("Image Browser Out"=w303:T1)  [unwired: 5 in, 4 out]
                n278 = call "IMAQ WindDraw"("Window Number (0...15)"=0, "Image"=w303) -> ()  [unwired: 8 in, 2 out]
                n279 = local read "Pra_Blk目录"() -> (w309:path)
                n280 = Concatenate Strings(w321, "_" ("字符串"), w314, ".bmp" ("字符串")) -> (w312:string)
                n281 = call "IMAQ Cast Image"("Image Type"=w310, "Image Dst"=w306, "Image Src"=w299) -> ("Image Dst Out"=w302:T1)  [unwired: 7 in, 1 out]
                n282 = Build Path(base path=w309, name or relative path=w312) -> (appended path=w311:path)
                n283 = call-poly "IMAQ Write File 2"("File Path"=w311, "Image"=w302) -> ()  [unwired: 8 in, 2 out]
              }
              n284 = local write "log"(w282) -> ()
            }
          }
        }
        frame Error {
          n285 = local write "开始/暂停"(TRUE ("开始/暂停")) -> ()
          n286 = One Button Dialog(message="blk exist, please change the file name" ("消息")) -> ()  [unwired: 1 in, 1 out]
        }
      }
      "block" <- w245
    }
    n287 = Array Size(array="Pra_stim ID") -> (size(s)=w214:i32)
    n288 = local write "Stimuli"(w214) -> ()
    n289 = property on="Pra_bin" class="Enum (严格)"("DisabledEnum"=w211) -> ()  [unwired: 2 in, 2 out]
    n290 = property on="SaveParameter" class="Bool"("DisabledEnum"=w211) -> ()  [unwired: 2 in, 2 out]
    n291 = property on="Pra_binType" class="Enum (严格)"("DisabledEnum"=w211) -> ()  [unwired: 2 in, 2 out]
    n292 = local read "停止循环"() -> (w220:bool)
  }
  n293 = local write "FrameWidth"(w20) -> ()
  n294 = local write "FrameHeight"(w19) -> ()
  n295 = node-c288() -> (w65:T15)
  n296 = timed-loop {
    tunnel: [w559] -> w60
    tunnel: [w581] -> w9
    tunnel: w17 -> [w560]
    tunnel: w5 -> [w580]
    tunnel: w6 -> [w579]
    tunnel: [w578] -> w45
    timing: w65 -> [_]
    timing-out: [_] -> w64
    tunnel: w41 -> [w569]
    tunnel: w13 -> [w564]
    tunnel: w36 -> [w574]
    tunnel: w32 -> [_]
    tunnel: w33 -> [w573]
    tunnel: w30 -> [w572]
    shift-right: [w567] -> _
    shift-left: 1 -> [w568]
    shift-right: [w566] -> _
    shift-left: w25 -> [w565]
    tunnel: w22 -> [w562]
    tunnel: w21 -> [w561]
    tunnel: w20 -> [w557]
    tunnel: w19 -> [w556]
    tunnel: "Pra_binType" -> [w555]
    shift-right: [w549] -> _
    shift-left: _ -> [w553]
    shift-right: [w550] -> _
    shift-left: _ -> [w548]
    tunnel: w14 -> [w547]
    shift-right: [w546] -> _
    shift-left: _ -> [w545]
    tunnel: [w544] -> w1
    i -> [w551]
    stop <- w575 stop-if-true
    n297 = node-c288() -> (→"循环持续时间":i64)  [unwired: 1 in]
    n298 = flat-sequence {
      frame #0 {
      }
      frame #1 {
        n299 = event shown="[3] \"LoadParameter\": 值改变" {
          selector: _ -> [_ _ _ _]
          dyn-events: _ -> [_ _ _ _]
          timeout: 0 -> [_ _ _ _]
          event Timeout {
            n300 = event-data() -> ()  [unwired: 1 in, 2 out]
          }
          event "停止": Value Change {
            n301 = event-data() -> ("NewVal"=w657:bool)  [unwired: 1 in, 1 out]
            n302 = case shown="真" w657 {
              selector: w657 -> [_ w659]
              tunnel: [FALSE w659] -> _
              frame False {
              }
              frame True {
                n303 = local write "开始/暂停"(w659) -> ()
                "停止循环" <- w659
              }
            }
          }
          event "SaveParameter": Value Change {
            n304 = event-data() -> ()  [unwired: 1 in, 1 out]
            n305 = call "文件对话框"("prompt"="SaveParameterTo", "pattern (all files)"="*.prmf", "pattern label"="Flowbit") -> ("selected path"=w661:path, "error out"=w663:errorcluster)  [unwired: 9 in, 2 out]
            n306 = case shown="无错误" w663 {
              tunnel: w661 -> [w666 _]
              frame No Error {
                n307 = control-ref of="本VI"() -> (w670:refnum<vi>)
                n308 = invoke class="VI" method="Ctrl Val.Get All"(reference=w670, "Controls"=TRUE ("输入控件")) -> ("Get All Control Values Variant"=w669:cluster{"Name":string, "Variant Data":variant}[])  [unwired: 2 in, 3 out]
                n309 = for {
                  tunnel: w669 -> [w674] mode=indexing
                  shift-right: [w673] -> w667
                  shift-left: cluster{"Name":string, "Variant Data":variant}[] [] -> [w672]
                  i -> [w671]
                  n310 = Unbundle By Name(w674) -> ("Name"=w679:string)
                  n311 = String Subset(string=w679, length (rest)=4 ("长度（剩余）")) -> (substring=w677:string)  [unwired: 1 in]
                  n312 = Equal?(x=w677, y="Pra_") -> (x = y?=w675:bool)
                  n313 = case shown="真" w675 {
                    tunnel: w674 -> [_ w684]
                    tunnel: [w680 w683] -> w673
                    tunnel: w672 -> [w680 w682]
                    tunnel: w671 -> [_ w681]
                    frame False {
                    }
                    frame True {
                      n314 = case shown="0" w681 {
                        tunnel: w684 -> [w686 w689]
                        tunnel: [w685 w688] -> w683
                        tunnel: w682 -> [_ w687]
                        frame 0 {
                          n315 = Build Array(w686) -> (w685:cluster{"Name":string, "Variant Data":variant}[])
                        }
                        frame 1, Default {
                          n316 = Build Array (concatenate)(w687, w689) -> (w688:cluster{"Name":string, "Variant Data":variant}[])
                        }
                      }
                    }
                  }
                }
                n317 = Write to Binary File(file (use dialog)=w666, data=w667) -> ()  [unwired: 4 in, 3 out]
              }
              frame Error {
              }
            }
          }
          event "LoadParameter": Value Change {
            n318 = event-data() -> ()  [unwired: 1 in, 1 out]
            n319 = call "文件对话框2"("prompt"="LoadParameter", "pattern (all files)"="*.prmf", "pattern label"="Flowbit") -> ("selected path"=w691:path, "error out"=w692:errorcluster)  [unwired: 9 in, 2 out]
            n320 = case shown="无错误" w692 {
              tunnel: w691 -> [w704 _]
              tunnel: [w700 _] -> w690
              frame No Error {
                n321 = Read from Binary File(5:cluster{"Name":string, "Variant Data":variant}[] [], 11:w704) -> (2:w701:cluster{"Name":string, "Variant Data":variant}[])  [unwired: 4 in, 3 out]
                n322 = control-ref of="本VI"() -> (w702:refnum<vi>)
                n323 = for {
                  tunnel: w702 -> [w710]
                  tunnel: w701 -> [w709] mode=indexing
                  tunnel: [w705] -> w700 mode=indexing
                  n324 = Unbundle By Name(w709) -> ("Name"=w708:string, "Variant Data"=w707:variant)
                  n325 = invoke class="VI" method="Ctrl Val.Set"(reference=w710, "Control Name"=w708, "Value"=w707) -> (error out=w706:errorcluster)  [unwired: 2 in, 4 out]
                  n326 = call <vilib>:"Clear Errors.vi"("error in (no error)"=w706) -> ("error out"=w705:errorcluster)  [unwired: 6 in]
                }
              }
              frame Error {
              }
            }
            n327 = flat-sequence {
              tunnel: w690 -> [_]
              frame #0 {
                n328 = Wait (ms)(milliseconds to wait=u32 20 ("等待时间（毫秒）")) -> ()  [unwired: 1 out]
              }
              frame #1 {
                n329 = local read "Pra_LED_Max_Voltage(V)"() -> (w697:dbl)
                n330 = local read "Pra_LED_COM"() -> (w699:refnum<visa-resource-name>)
                n331 = call <userlib>:"GWPS320x Application Example.vi"("OVP(V) (0.000)"=w697, "Output State (F:Off)"=TRUE, "VISA session"=w699) -> ()  [unwired: 5 in, 4 out]
              }
            }
          }
        }
      }
    }
    n332 = Get Queue Status(queue=w564) -> (queue out=w563:refnum<queue>, # elements in queue=→"队列中元素数量":i32)  [unwired: 2 in, 6 out]
    n333 = case shown="\"2*2\"" "Pra_bin" {
      tunnel: w562 -> [_ w643]
      tunnel: w561 -> [_ w638]
      tunnel: w560 -> [w636 w642]
      tunnel: [w636 w641] -> w559
      tunnel: w557 -> [_ w647]
      tunnel: w556 -> [_ w644]
      tunnel: w555 -> [_ w637]
      frame "1*1", Default {
      }
      frame "2*2" {
        n334 = Divide(x=w647, y=2) -> (x/y=w640:dbl)
        n335 = Divide(x=w644, y=2) -> (x/y=w639:dbl)
        n336 = local write "FrameWidth"(w640) -> ()
        n337 = case shown="\"Resample\"" w637 {
          tunnel: w643 -> [_ w654]
          tunnel: w642 -> [w649 w655]
          tunnel: [w648 w651] -> w641
          tunnel: w640 -> [_ w653]
          tunnel: w639 -> [_ w652]
          tunnel: w638 -> [_ w650]
          frame "Extract", Default {
            n338 = call "Bin2.vi"("Image Src"=w649) -> ("Image"=w648:T1)  [unwired: 10 in]
          }
          frame "Resample" {
            n339 = call "IMAQ Resample"("X Resolution"=w653, "Y Resolution"=w652, "Interpolation Type"=w650, "Image Dst"=w654, "Image Src"=w655) -> ("Image Dst Out"=w651:T1)  [unwired: 5 in, 1 out]
          }
        }
        n340 = local write "FrameHeight"(w639) -> ()
      }
    }
    n341 = local read "Recording"() -> (w549:bool)
    n342 = case shown="真" w549 {
      tunnel: w563 -> [w582 w594]
      tunnel: w559 -> [_ w599]
      tunnel: w569 -> [_ w598]
      tunnel: w568 -> [_ w590]
      tunnel: [1 w595] -> w567
      tunnel: w565 -> [_ w591]
      tunnel: [u32[][] [] w593] -> w566
      tunnel: [w583 w587] -> w546
      tunnel: w545 -> [_ w588]
      tunnel: [w582 w586] -> w544
      frame False {
        n343 = local read "Pra_FramesPerStim"() -> (w583:i64)
      }
      frame True {
        n344 = call "IMAQ Copy"("Image Dst"=w598, "Image Src"=w599) -> ("Image Dst Out"=w597:T1)  [unwired: 4 in, 1 out]
        n345 = call "IMAQ ImageToArray"("Image"=w597) -> ("Image Pixels (I16)"=w592:i16[][])  [unwired: 3 in, 4 out]
        n346 = Greater?(x="Pra_FrameBin", y=w590) -> (0:w596:bool)
        n347 = case shown="假" w596 {
          tunnel: w590 -> [_ w620]
          tunnel: [1 w619] -> w595
          tunnel: w594 -> [w609 w617]
          tunnel: [u32[][] [] w622] -> w593
          tunnel: w592 -> [w608 w624]
          tunnel: w591 -> [w607 w623]
          tunnel: w590 -> [_ w621]
          tunnel: "Pra_FrameBin" -> [w604 _]
          tunnel: w588 -> [w603 w618]
          tunnel: [w601 w618] -> w587
          tunnel: [w600 w617] -> w586
          frame False {
            n348 = case shown="0, 默认" w604 {
              tunnel: w608 -> [w614 w616]
              tunnel: w607 -> [w613 _]
              tunnel: [w612 w615] -> w605
              frame 0, Default {
                n349 = Add(x=w614, y=w613) -> (x+y=w612:u32[][])
              }
              frame 1 {
                n350 = To Unsigned Long Integer(number=w616) -> (unsigned 32bit integer=w615:u32[][])
              }
            }
            n351 = Decrement(x=w603) -> (x-1=w601:i64)
            n352 = Less Or Equal To 0?(x=w601) -> (x <= 0?=w602:bool)
            n353 = case shown="真" w602 {
              frame False {
              }
              frame True {
                n354 = local write "Recording"(FALSE ("Recording")) -> ()
              }
            }
            n355 = Enqueue Element(queue=w609, element=w605) -> (queue out=w600:refnum<queue>)  [unwired: 2 in, 2 out]
          }
          frame True {
            n356 = case shown="1" w621 {
              tunnel: w624 -> [w625 w628]
              tunnel: w623 -> [_ w627]
              tunnel: [w625 w626] -> w622
              frame 1 {
              }
              frame 0, Default {
                n357 = Add(x=w628, y=w627) -> (x+y=w626:u32[][])
              }
            }
            n358 = Increment(x=w620) -> (x+1=w619:i32)
          }
        }
      }
    }
    n359 = Not Equal?(x=w549, y=w553) -> (x != y?=w552:bool)
    n360 = case shown="假" "热图" {
      tunnel: w574 -> [w717 w725]
      tunnel: w559 -> [w711 w723]
      tunnel: [w711 w722] -> w571
      tunnel: w573 -> [_ w720]
      tunnel: w572 -> [_ w719]
      tunnel: w547 -> [w715 _]
      frame False {
        w716 = T4 0 items=["Grayscale (U8)", "Grayscale (I16)", "Grayscale (SGL)", "Complex (CSG)", "RGB (U32)", "HSL (U32)", "RGB (U64)", "Grayscale (U16)"] ("Image Type")
        n361 = call "IMAQ Copy"("Image Dst"=w717, "Image Src"=w711) -> ("Image Dst Out"=w714:T1)  [unwired: 4 in, 1 out]
        n362 = call "IMAQ Divide"("Image Src A"=w714, "Constant"=sgl 16.0, "Image Dst"=w714) -> ("Image Dst Out"=w712:T1)  [unwired: 4 in, 1 out]
        n363 = call "IMAQ Cast Image"("Image Type"=w716, "Image Dst"=w715, "Image Src"=w712) -> ()  [unwired: 7 in, 2 out]
      }
      frame True {
        w721 = T4 4 items=["Grayscale (U8)", "Grayscale (I16)", "Grayscale (SGL)", "Complex (CSG)", "RGB (U32)", "HSL (U32)", "RGB (U64)", "Grayscale (U16)"] ("Image Type")
        n364 = call "IMAQ Copy"("Image Dst"=w725, "Image Src"=w723) -> ("Image Dst Out"=w724:T1)  [unwired: 4 in, 1 out]
        n365 = call "IMAQ Divide"("Image Src A"=w724, "Constant"=sgl 256.0, "Image Dst"=w724) -> ("Image Dst Out"=w718:T1)  [unwired: 4 in, 1 out]
        n366 = call "IMAQ Cast Image"("Image Type"=w721, "Lookup Table"=w719, "Image Dst"=w720, "Image Src"=w718) -> ("Image Dst Out"=w722:T1)  [unwired: 6 in, 1 out]
      }
    }
    "Image 2" <- w571
    n367 = case shown="真" w552 {
      tunnel: w551 -> [_ w630]
      tunnel: [w629 w630] -> w550
      tunnel: w548 -> [w629 w631]
      tunnel: w549 -> [_ w632]
      tunnel: w548 -> [_ _]
      frame False {
      }
      frame True {
        n368 = case shown="假" w632 {
          tunnel: w631 -> [w634 _]
          tunnel: w630 -> [w633 _]
          frame False {
            n369 = Subtract(x=w633, y=w634) -> (x-y=→"grabLoop":i32)
          }
          frame True {
          }
        }
      }
    }
    n370 = local read "停止循环"() -> (w575:bool)
    n371 = call <vilib>:"Wait For Frame.vi"("error in (no error)"=w580, "Timeout (mS)"=u32 5000, "RefBrdIn"=w579) -> ("error out"=w581:errorcluster, "RefBrdOut"=w578:u32)  [unwired: 7 in]
    n372 = node-c288() -> ()  [unwired: 1 in, 1 out]
  }
  n373 = node-c288(w64) -> ()  [unwired: 1 out]
  n374 = call "IMAQ WindClose"("Close All Windows (False)"=TRUE, "error in (no error)"=w9) -> ("error out"=w8:errorcluster)  [unwired: 4 in]
  n375 = call <vilib>:"Stop.vi"("error in (no error)"=w8, "Image In"=w60, "RefBrdIn"=w45) -> ("error out"=w56:errorcluster, "Image"=w59:T1, "RefBrdOut"=w44:u32)  [unwired: 6 in]
  n376 = call <vilib>:"Cleanup.vi"("error in (no error)"=w56, "Image In"=w59, "RefBrdIn"=w44) -> ("error out"=w57:errorcluster, "Image"=w58:T1, "RefBrdOut"=w43:u32)  [unwired: 6 in]
  n377 = call <vilib>:"Close.vi"("error in (no error)"=w57, "RefBrdIn"=w43) -> ("error out"=w42:errorcluster)  [unwired: 8 in, 1 out]
  n378 = call "Imaq Dispose"("Image"=w58, "error in (no error)"=w42) -> ("error out"=w3:errorcluster)  [unwired: 4 in]
  n379 = flat-sequence {
    tunnel: w3 -> [w732]
    tunnel: [w731] -> w2
    tunnel: w1 -> [w730]
    tunnel: w2 -> [w735]
    frame #0 {
      n380 = Flush Queue(queue=w730, error in (no error)=w732) -> (error out=w731:errorcluster)  [unwired: 2 out]
    }
    frame #1 {
      w733 = 0.0 ("Output Voltage (V) (0.0)")
      n381 = local read "Pra_LED_COM"() -> (w734:refnum<visa-resource-name>)
      n382 = call <userlib>:"GWPS320x Configure Voltage - Current.vi"("VISA session"=w734, "Output Voltage (V) (0.0)"=w733, "Output Current (A) (0.0)"=w733, "error in (no error)"=w735) -> ()  [unwired: 10 in, 2 out]
    }
    frame #2 {
      n383 = Stop(stop? (T)=TRUE ("停止？(T)")) -> ()
    }
  }
